vi "Insert Autostart Step.vi"(0 "VISA resource name":refnum<visa-resource-name>, 1 "Unit Address (1)":i16=1, 2 "Date Or Day (0: Date)":u16(ring) items=["Date", "Day"], 3 "Day Of Week (0: Every Day)":u16(ring) items=["Every Day", "Sunday", "Monday", "Tuesday", "Wednesday", "Thursday", "Friday", "Saturday"], 5 "Current Step Number (1)":i16=1, 7 "Date (1; 1; 2004)":i16[](array[numeric])=[1, 1, 2004], 9 "Time (0; 0; 0)":i16[](array[numeric])=[0, 0, 0], 11 "error in (no error)":errorcluster {"code" format="%.0x"}) -> (4 "VISA resource name out":refnum<visa-resource-name>, 15 "error out":errorcluster {"code" format="%.0x"})   [LabVIEW 2010]
doc: "This VI inserts the autostart step."
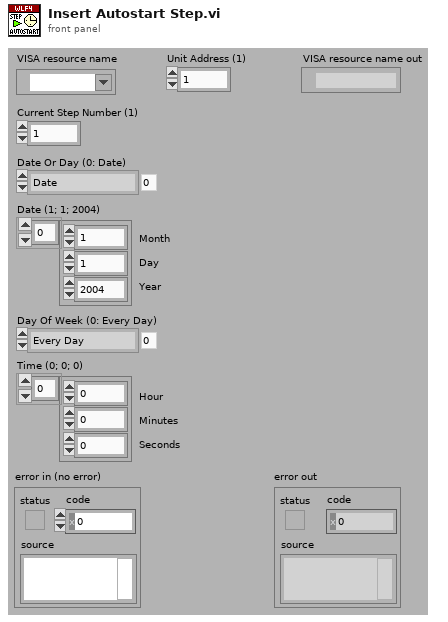
[diagram p1: front panel]
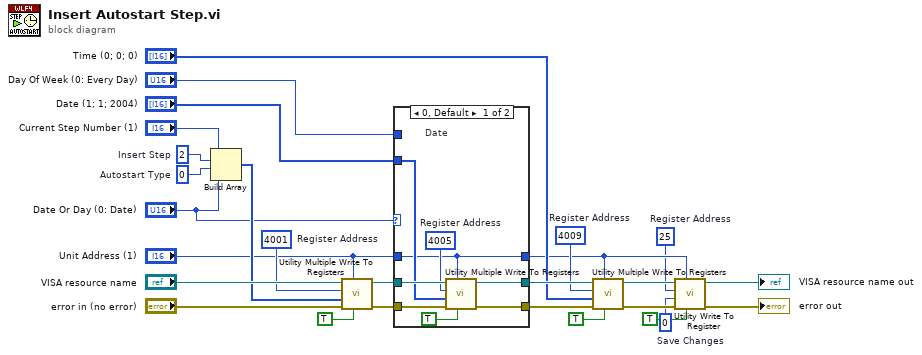
[diagram p0: block diagram]
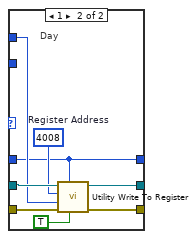
[diagram p2: hidden frame]
diagram:
  w5 = u16 2  # Insert Step
  w6 = i16 0  # Save Changes
  w7 = u16 25  # Register Address
  w13 = u16 4009  # Register Address
  w22 = u16 0  # Autostart Type
  w25 = u16 4001  # Register Address
  n1 = Build Array("Current Step Number (1)", w5, w22, "Date Or Day (0: Date)") -> (w23:u16[])
  n2 = call "Utility Multiple Write To Registers.vi"("Direct Action?"=TRUE, "Unit Address (1)"="Unit Address (1)", "error in (no error)"="error in (no error)", "Array Of Data"=w23, "Register Address (0)"=w25, "VISA resource name"="VISA resource name") -> ("error out"=w20:errorcluster, "VISA resource name out"=w21:refnum<visa-resource-name>)  [unwired: 4 in]
  n3 = case shown="0, Default" "Date Or Day (0: Date)" {
    tunnel: w21 -> [w33 w40]
    tunnel: w20 -> [w35 w43]
    tunnel: [w34 w42] -> w16
    tunnel: [w32 w41] -> w15
    tunnel: "Unit Address (1)" -> [w29 w37]
    tunnel: "Date (1; 1; 2004)" -> [w31 _]
    tunnel: "Day Of Week (0: Every Day)" -> [_ w39]
    tunnel: [w29 w37] -> w8
    frame 0, Default {
      w30 = u16 4005  # Register Address
      # "Date"
      n4 = call "Utility Multiple Write To Registers.vi"("Direct Action?"=TRUE, "Unit Address (1)"=w29, "error in (no error)"=w35, "Array Of Data"=w31, "Register Address (0)"=w30, "VISA resource name"=w33) -> ("error out"=w34:errorcluster, "VISA resource name out"=w32:refnum<visa-resource-name>)  [unwired: 4 in]
    }
    frame 1 {
      w38 = u16 4008  # Register Address
      # "Day"
      n5 = call "Utility Write To Register.vi"("Direct Action?"=TRUE, "Unit Address (1)"=w37, "error in (no error)"=w43, "Data (0)"=w39, "Register Address (0)"=w38, "VISA resource name"=w40) -> ("error out"=w42:errorcluster, "VISA resource name out"=w41:refnum<visa-resource-name>)  [unwired: 4 in]
    }
  }
  n6 = call "Utility Multiple Write To Registers.vi"("Direct Action?"=TRUE, "Unit Address (1)"=w8, "error in (no error)"=w16, "Array Of Data"="Time (0; 0; 0)", "Register Address (0)"=w13, "VISA resource name"=w15) -> ("error out"=w12:errorcluster, "VISA resource name out"=w9:refnum<visa-resource-name>)  [unwired: 4 in]
  n7 = call "Utility Write To Register.vi"("Direct Action?"=TRUE, "Unit Address (1)"=w8, "error in (no error)"=w12, "Data (0)"=w6, "Register Address (0)"=w7, "VISA resource name"=w9) -> ("error out"=→"error out":errorcluster, "VISA resource name out"=→"VISA resource name out":refnum<visa-resource-name>)  [unwired: 4 in]
